vi "New User Dialog.vi"(0 "Enable":bool=TRUE, 5 "error in (no error)":errorcluster) -> (15 "Access Level":T1 items=["Admin"=0, "User"=1, "Guest"=10], 16 "Password":string, 17 "Username":string, 18 "OK":bool, 19 "error out":errorcluster)   [LabVIEW 2016, in "UserPwd DB.lvlib" / "UserPwd DB Configuration.lvclass"]
doc: "Displays a standard dialog box that prompts users to enter information, such as a user name and password.\n--------------------\n\nThis Express VI is configured as follows:\n\nMessage to Display to the User:Create a new user\nThe inputs are: \nText Entry Box: Username\nText Entry Box: Password\nNumber: Access Level"
uses:
  <userlib>/Common Components/UserPwd DB/UserPwd DB Config/UserPwd DB Configuration.lvclass
  <userlib>/Common Components/UserPwd DB/UserPwd DB Config/Access Level.ctl
panel:
  in  "Access Level":T1=1 items=["Admin"=0, "User"=1, "Guest"=10]
  in  "Password":string
  in  "Username (max 15 characters)":string caption="Username"
  out "String":string="Create a new user"
  in  "Cancel":bool
  in  "OK2":bool
  in  "OK1":bool
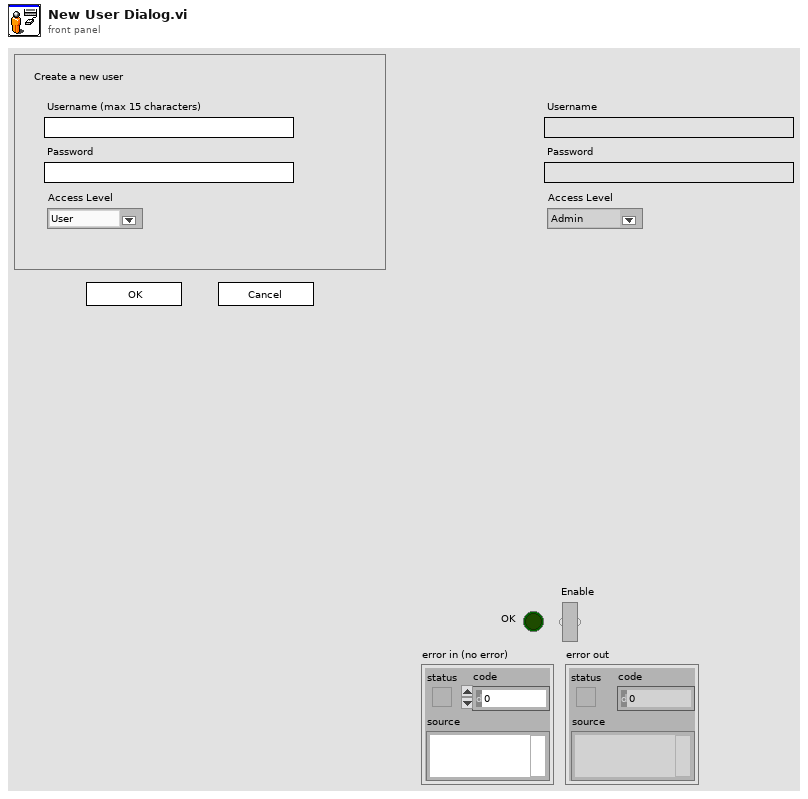
[diagram p1: front panel]
types:
  T1 = typedef "UserPwd DB.lvlib/UserPwd DB Configuration.lvclass/Access Level.ctl" = u16
  T2 = cluster{"Input Name":string, "Input Data Type":i32}[]
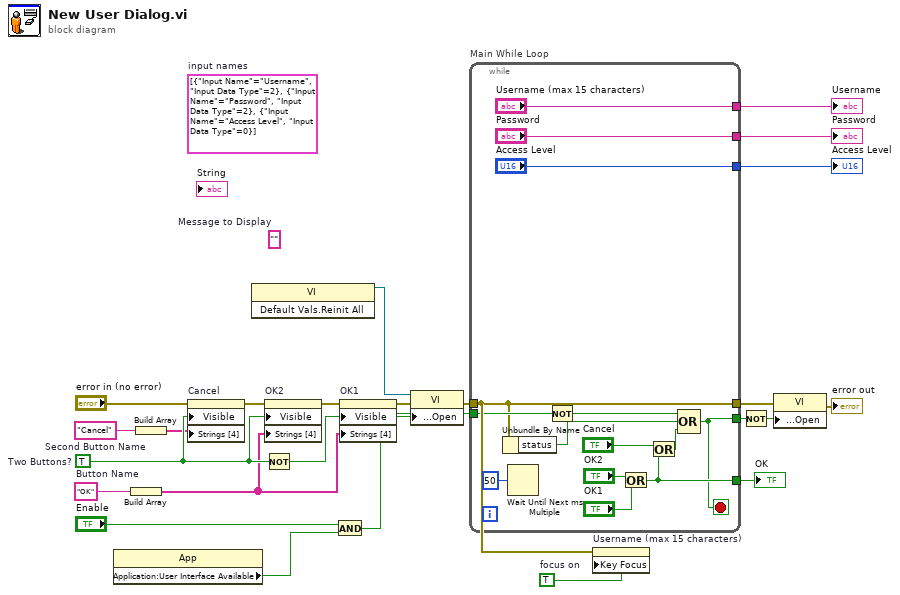
[diagram p0: block diagram]
diagram:
  w3 = TRUE  # focus on
  (unwired) T2 [{"Input Name"="Username", "Input Data Type"=2}, {"Input Name"="Password", "Input Data Type"=2}, {"Input Name"="Access Level", "Input Data Type"=0}]  # input names
  w16 = "Cancel"  # Second Button Name
  w14 = "OK"  # Button Name
  (unwired) ""  # Message to Display
  w24 = TRUE  # Two Buttons?
  n1 = property class="App"() -> ("Application:User Interface Available"=w6:bool)  [unwired: 2 in, 2 out]
  n2 = Build Array(w14) -> (w15:string[])
  n3 = Build Array(w16) -> (w17:string[])
  n4 = property on="Cancel" class="Bool"(error in="error in (no error)", "Visible"=w24, "Strings [4]"=w17) -> (error out=w21:errorcluster)  [unwired: 1 in, 1 out]
  n5 = invoke class="VI" method="Default Vals.Reinit All"() -> (reference out=w5:refnum<vi>)  [unwired: 3 in, 2 out]
  n6 = Not(x=w24) -> (.not. x?=w22:bool)
  n7 = property on="OK2" class="Bool"(error in=w21, "Visible"=w24, "Strings [4]"=w15) -> (error out=w20:errorcluster)  [unwired: 1 in, 1 out]
  n8 = And(x="Enable", y=w6) -> (x .and. y?=w7:bool)
  n9 = property on="OK1" class="Bool"(error in=w20, "Visible"=w22, "Strings [4]"=w15) -> (error out=w13:errorcluster)  [unwired: 1 in, 1 out]
  n10 = property class="VI"(reference=w5, error in=w13, "Front Panel Window:Open"=w7) -> (error out=w12:errorcluster)  [unwired: 1 out]
  n11 = while "Main While Loop" {
    tunnel: [w35] -> w23
    tunnel: w7 -> [w33]
    tunnel: [w31] -> w18
    tunnel: w12 -> [w30]
    tunnel: [w30] -> w10
    tunnel: ["Username (max 15 characters)"] -> w4
    tunnel: ["Password"] -> w2
    tunnel: ["Access Level"] -> w1
    stop <- w31 stop-if-true
    n12 = Unbundle By Name(w30) -> ("status"=w28:bool)
    n13 = Wait Until Next ms Multiple(millisecond multiple=u32 50) -> ()  [unwired: 1 out]
    n14 = Not(x=w33) -> (.not. x?=w32:bool)
    n15 = Or(x="OK2", y="OK1") -> (x .or. y?=w35:bool)
    n16 = Or(x="Cancel", y=w35) -> (x .or. y?=w29:bool)
    n17 = Compound Arithmetic op=OR(w32, w28, w29) -> (w31:bool)
  }
  "OK" <- w23
  "Username" <- w4
  "Password" <- w2
  "Access Level" <- w1
  n18 = property on="Username (max 15 characters)" class="Str"(error in=w12, "Key Focus"=w3) -> ()  [unwired: 1 in, 2 out]
  n19 = Not(x=w18) -> (.not. x?=w19:bool)
  n20 = property class="VI"(error in=w10, "Front Panel Window:Open"=w19) -> (error out=→"error out":errorcluster)  [unwired: 1 in, 1 out]
